vi "Get Temp Control--Accessor.vi"(8 "error in (no error)":errorcluster, 11 "Simulated Thermal Process Controller in":refnum<class "Simulated Thermal Process Controller.lvclass">) -> (0 "error out":errorcluster, 2 "Temp Control":bool, 3 "Simulated Thermal Process Controller out":refnum<class "Simulated Thermal Process Controller.lvclass">)   [LabVIEW 2024, in "Simulated Thermal Process Controller.lvclass"]
uses:
  Simulated Thermal Process Controller.lvclass
  Simulated Thermal Process Controller.lvclass/Simulated Thermal Process Controller.ctl
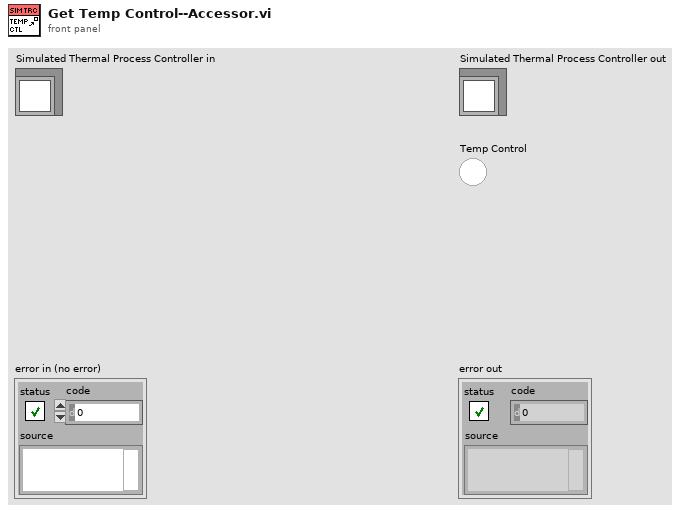
[diagram p1: front panel]
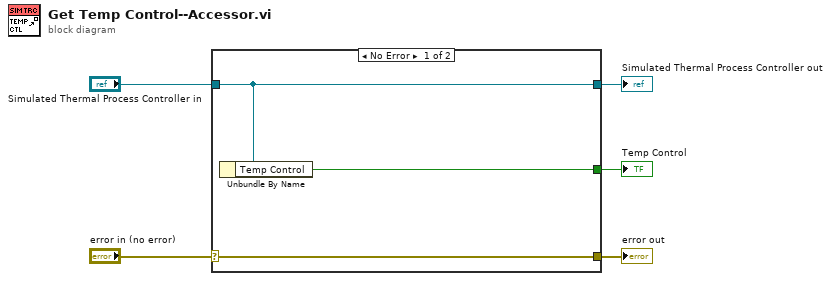
[diagram p0: block diagram]
diagram:
  n1 = case shown="No Error" "error in (no error)" {
    selector: "error in (no error)" -> [w8 w9]
    tunnel: [w8 w9] -> w4
    tunnel: [w7 w10] -> w2
    tunnel: "Simulated Thermal Process Controller in" -> [w7 w10]
    tunnel: [w6 _] -> w1
    frame No Error {
      n2 = Unbundle By Name(w7) -> ("Temp Control"=w6:bool)
    }
    frame Error {
    }
  }
  "error out" <- w4
  "Simulated Thermal Process Controller out" <- w2
  "Temp Control" <- w1
